vi "RELAYS Read Optos.vi"(8 "error in (no error)":errorcluster, 10 "Dev Addr":u8=1, 11 "VISA resource name":refnum<visa-resource-name>) -> (0 "error out":errorcluster, 1 "Optos Status":bool[](array[boolean]), 2 "ack":string, 3 "VISA resource name out":refnum<visa-resource-name>)   [LabVIEW 2016, in "MB _relays.lvlib"]
uses:
  MB _relays.lvlib
  private/gen MB frame -Read optocoupler input status.vi
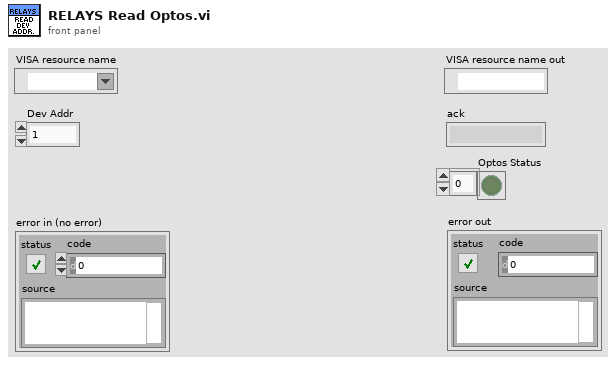
[diagram p1: front panel]
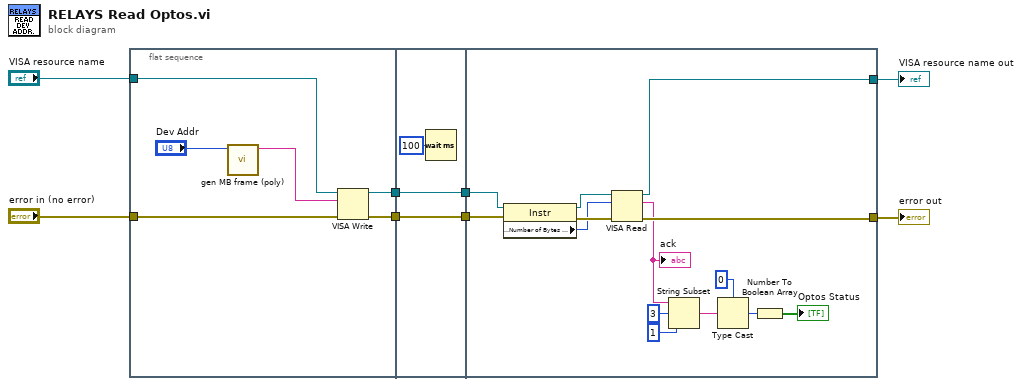
[diagram p0: block diagram]
diagram:
  n1 = flat-sequence {
    tunnel: "error in (no error)" -> [w11]
    tunnel: "VISA resource name" -> [w10]
    tunnel: [w14] -> w4
    tunnel: [w13] -> w3
    tunnel: w4 -> [w17]
    tunnel: w3 -> [w16]
    tunnel: [w17] -> w2
    tunnel: [w16] -> w1
    tunnel: [w25] -> w7
    tunnel: [w26] -> w8
    tunnel: w2 -> [w30]
    tunnel: w1 -> [w31]
    frame #0 {
      n2 = call-poly "gen MB frame (poly).vi"("Dev Addr"="Dev Addr") -> ("MB frame"=w12:string)  [unwired: 10 in]
      n3 = VISA Write(VISA resource name=w10, write buffer=w12, error in (no error)=w11) -> (VISA resource name out=w14:refnum<visa-resource-name>, error out=w13:errorcluster)  [unwired: 1 out]
    }
    frame #1 {
      n4 = Wait (ms)(milliseconds to wait=u32 100) -> ()  [unwired: 1 out]
    }
    frame #2 {
      n5 = property class="Instr"(reference=w30, error in=w31) -> (reference out=w28:refnum<visa-resource-name>, error out=w29:errorcluster, "Serial Settings:Number of Bytes at Serial Port"=w27:u32)
      n6 = VISA Read(VISA resource name=w28, byte count=w27, error in (no error)=w29) -> (VISA resource name out=w26:refnum<visa-resource-name>, read buffer=w24:string, error out=w25:errorcluster)  [unwired: 1 out]
      "ack" <- w24
      n7 = String Subset(string=w24, offset (0)=3, length (rest)=1 ("length (rest)")) -> (substring=w21:string)
      n8 = Type Cast(type=u8 0, x=w21) -> (*(type *) &x=w19:u8)
      n9 = Number To Boolean Array(number=w19) -> (Boolean array=→"Optos Status":bool[])
    }
  }
  "VISA resource name out" <- w8
  "error out" <- w7
